vi "colab.vi"() -> ()   [LabVIEW 2021]
uses:
  <vilib>/userdefined/High Color/IMAQdx.ctl
  <vilib>/vision/driver/NI_Vision_Acquisition_Software.lvlib
panel:
  in  "stop 2":bool
  in  "servo":bool
  out "error out 2":errorcluster
  in  "Image Name 2":string="untitled"
  out "Image":T1(plugin-control)
  in  "Robot IP Address":string
  in  "Port 2":u16=1024 min=1024
  in  "Speed":dbl(slide) scale=0.0..255.0
  in  "stop":bool
  out "Connected LED":bool
  in  "Tien":bool
  in  "Lui":bool
  in  "Trai":bool
  in  "Phai":bool
  out "Trang thai ket noi":string
  out "Lenh da gui":string
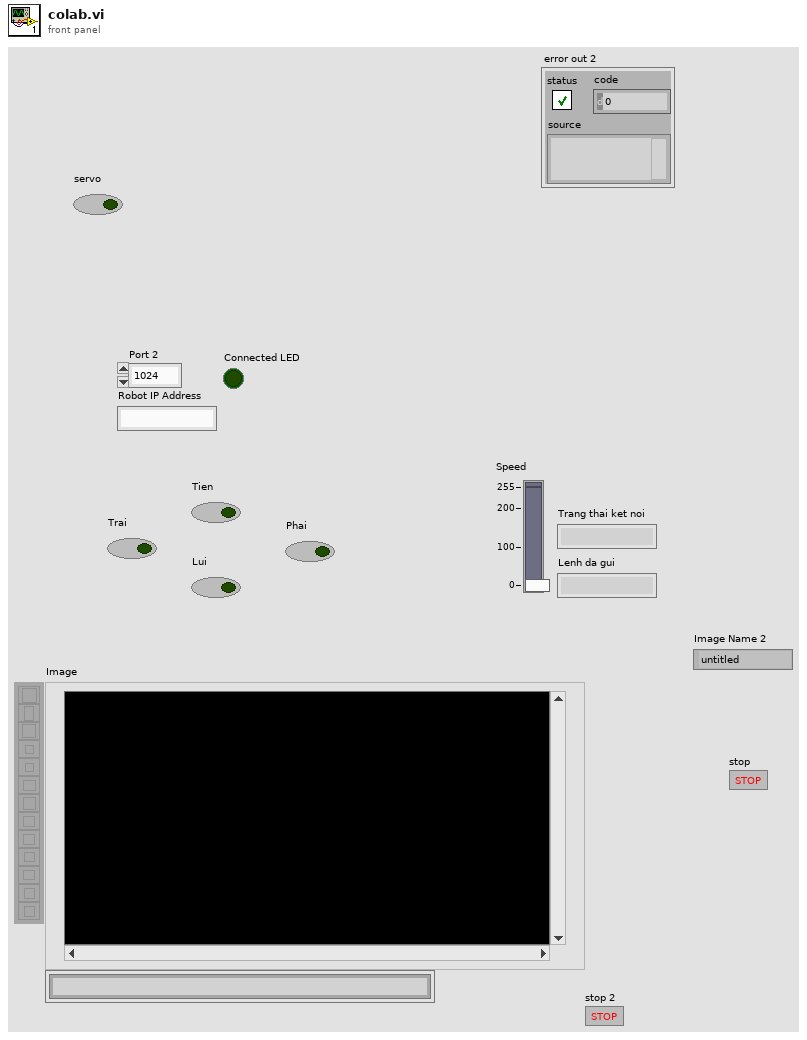
[diagram p1: front panel]
types:
  T1 = typedef "IMAQ Image.ctl" = refnum<image>
  T2 = typedef "IMAQdx.ctl" = refnum<k21>
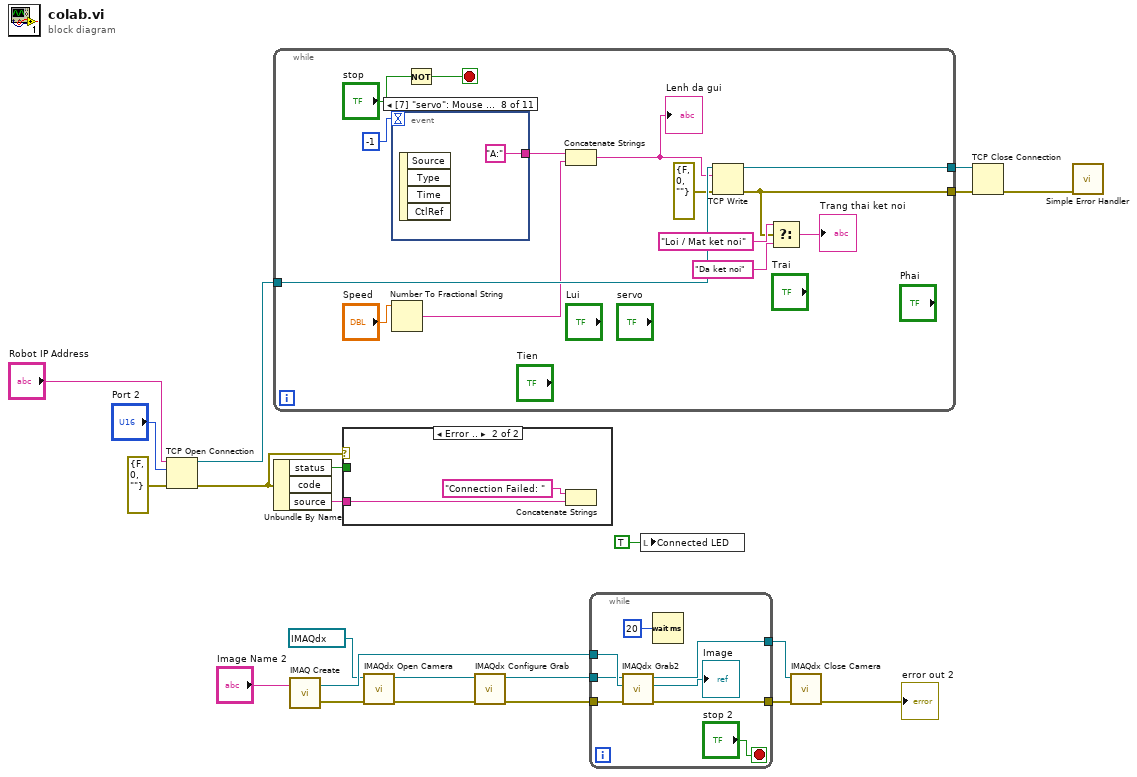
[diagram p0: block diagram]
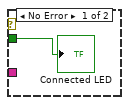
[diagram p2: hidden frame]
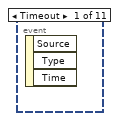
[diagram p3: hidden frame]
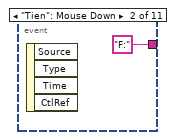
[diagram p4: hidden frame]
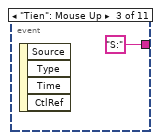
[diagram p5: hidden frame]
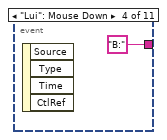
[diagram p6: hidden frame]
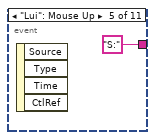
[diagram p7: hidden frame]
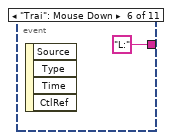
[diagram p8: hidden frame]
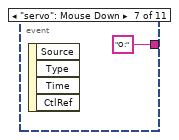
[diagram p9: hidden frame]
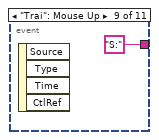
[diagram p10: hidden frame]
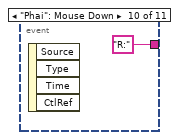
[diagram p11: hidden frame]
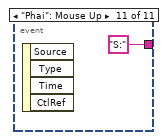
[diagram p12: hidden frame]
diagram:
  n1 = TCP Open Connection(address="Robot IP Address", remote port or service name="Port 2", error in (no error)=errorcluster {"status"=FALSE, "code"=0, "source"=""}) -> (connection ID=w15:refnum<k5>, error out=w14:errorcluster)  [unwired: 2 in]
  n2 = while {
    tunnel: w15 -> [w35]
    tunnel: [w31] -> w16
    tunnel: [w23] -> w17
    stop <- w32 stop-if-true
    n3 = event shown="[7] \"servo\": Mouse Up" {
      selector: _ -> [_ _ _ _ _ _ _ _ _ _ _]
      dyn-events: _ -> [_ _ _ _ _ _ _ _ _ _ _]
      timeout: -1 -> [_ _ _ _ _ _ _ _ _ _ _]
      tunnel: [_ "F:" ("data in") "S:" ("data in") "B:" ("data in") "S:" ("data in") "L:" ("data in") "O:" ("data in") "A:" ("data in") "S:" ("data in") "R:" ("data in") "S:" ("data in")] -> w25
      event Timeout {
        n4 = event-data() -> ()  [unwired: 1 in, 3 out]
      }
      event "Tien": Mouse Down {
        n5 = event-data() -> ()  [unwired: 1 in, 4 out]
      }
      event "Tien": Mouse Up {
        n6 = event-data() -> ()  [unwired: 1 in, 4 out]
      }
      event "Lui": Mouse Down {
        n7 = event-data() -> ()  [unwired: 1 in, 4 out]
      }
      event "Lui": Mouse Up {
        n8 = event-data() -> ()  [unwired: 1 in, 4 out]
      }
      event "Trai": Mouse Down {
        n9 = event-data() -> ()  [unwired: 1 in, 4 out]
      }
      event "servo": Mouse Down {
        n10 = event-data() -> ()  [unwired: 1 in, 4 out]
      }
      event "servo": Mouse Up {
        n11 = event-data() -> ()  [unwired: 1 in, 4 out]
      }
      event "Trai": Mouse Up {
        n12 = event-data() -> ()  [unwired: 1 in, 4 out]
      }
      event "Phai": Mouse Down {
        n13 = event-data() -> ()  [unwired: 1 in, 4 out]
      }
      event "Phai": Mouse Up {
        n14 = event-data() -> ()  [unwired: 1 in, 4 out]
      }
    }
    n15 = Number To Fractional String(number="Speed") -> (F-format string=w26:string)  [unwired: 3 in]
    n16 = Not(x="stop") -> (.not. x?=w32:bool)
    n17 = Concatenate Strings "Concatenate Strings"(w25, w26) -> (w24:string)
    "Lenh da gui" <- w24
    n18 = TCP Write(connection ID=w35, data in=w24, error in (no error)=errorcluster {"status"=FALSE, "code"=0, "source"=""}) -> (connection ID out=w31:refnum<k5>, error out=w23:errorcluster)  [unwired: 1 in, 1 out]
    n19 = Select(t="Loi / Mat ket noi", s=w23, f="Da ket noi") -> (s? t:f=→"Trang thai ket noi":string)
  }
  n20 = Unbundle By Name(w14) -> ("status"=w21:bool, "source"=w20:string)  [unwired: 1 out]
  n21 = call "IMAQ Create"("Image Name"="Image Name 2") -> ("New Image"=w11:T1, "error out"=w10:errorcluster)  [unwired: 4 in]
  n22 = case shown="Error .." w14 {
    tunnel: w20 -> [_ w48]
    tunnel: w21 -> [w47 _]
    frame No Error {
      "Connected LED" <- w47
    }
    frame Error {
      n23 = Concatenate Strings("Connection Failed: " ("string"), w48) -> ()  [unwired: 1 out]
    }
  }
  n24 = call <vilib>:"IMAQdx Open Camera.vi"("error in"=w10, "Session In"=T2 "cam0") -> ("error out"=w9:errorcluster, "Session Out"=w6:T2)  [unwired: 8 in]
  n25 = call <vilib>:"IMAQdx Configure Grab.vi"("error in"=w9, "Session In"=w6) -> ("error out"=w8:errorcluster, "Session Out"=w5:T2)  [unwired: 8 in]
  n26 = while {
    tunnel: w11 -> [w54]
    tunnel: w8 -> [w56]
    tunnel: w5 -> [w53]
    tunnel: [w55] -> w3
    tunnel: [w51] -> w1
    stop <- "stop 2" stop-if-true
    n27 = call <vilib>:"IMAQdx Grab2.vi"("error in"=w56, "Image In"=w54, "Session In"=w53) -> ("error out"=w55:errorcluster, "Image Out"=→"Image":T1, "Session Out"=w51:T2)  [unwired: 5 in, 1 out]
    n28 = Wait (ms)(milliseconds to wait=u32 20) -> ()  [unwired: 1 out]
  }
  n29 = local write "Connected LED"(TRUE) -> ()
  n30 = call <vilib>:"IMAQdx Close Camera.vi"("error in"=w3, "Session In"=w1) -> ("error out"=→"error out 2":errorcluster)  [unwired: 9 in]
  n31 = TCP Close Connection(connection ID=w16, error in (no error)=w17) -> (error out=w22:errorcluster)  [unwired: 1 in, 1 out]
  n32 = call <vilib>:"Simple Error Handler.vi"("error in (no error)"=w22) -> ()  [unwired: 4 in, 5 out]
